vi "RTS Server Send Data.vi"(4 "Skip Data Send":bool, 6 "error in (no error)":errorcluster, 8 "error IO":errorcluster, 10 "Send Data":string[][](array[string]), 11 "TCP Network Connection in":refnum<k5>) -> (0 "error out":errorcluster, 1 "Boolean":bool, 3 "TCP Network Connection out":refnum<k5>)   [LabVIEW 2016]
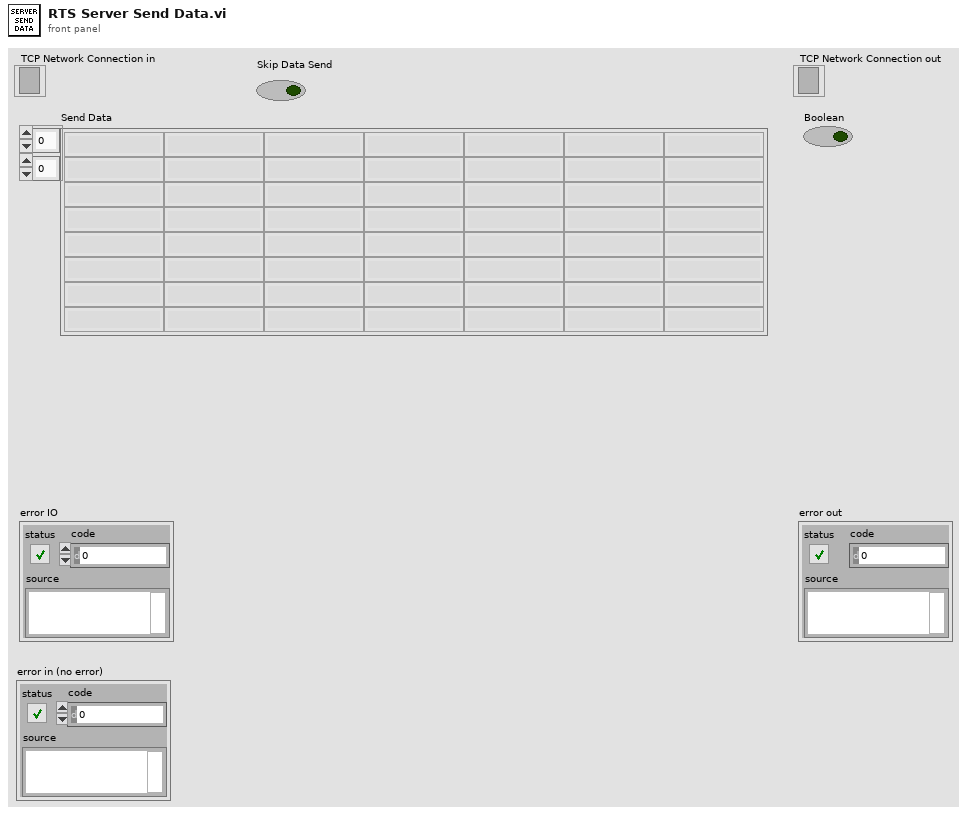
[diagram p1: front panel]
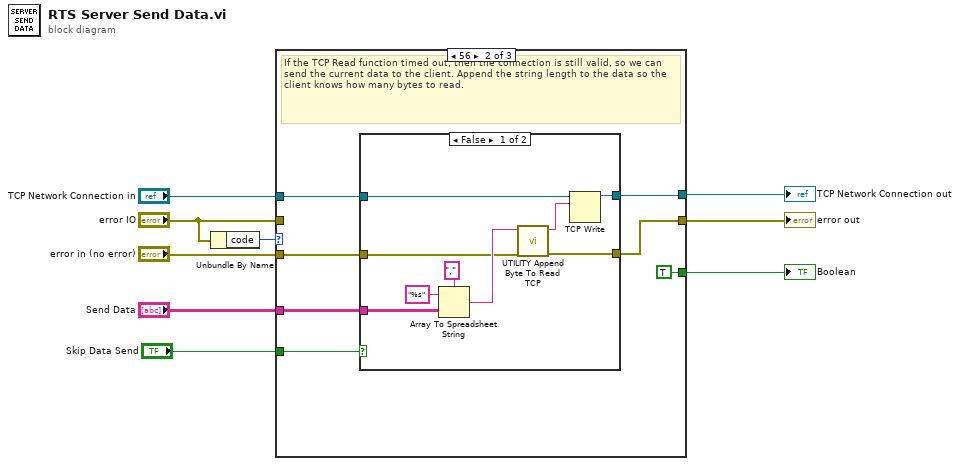
[diagram p0: block diagram]
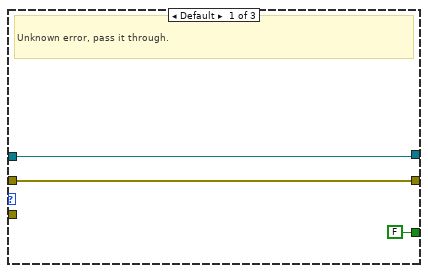
[diagram p2: hidden frame]
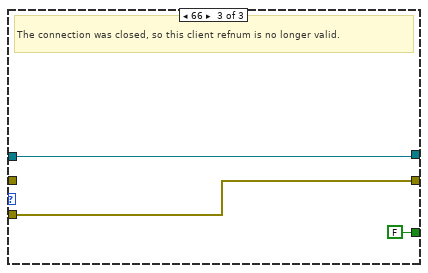
[diagram p4: hidden frame]
diagram:
  n1 = Unbundle By Name("error IO") -> ("code"=w8:i32)
  n2 = case shown="56" w8 {
    tunnel: "error IO" -> [w12 _ _]
    tunnel: [w12 w18 w33] -> w3
    tunnel: "error in (no error)" -> [_ w19 w33]
    tunnel: "TCP Network Connection in" -> [w10 w17 w31]
    tunnel: [w10 w16 w31] -> w6
    tunnel: [FALSE TRUE FALSE] -> w7
    tunnel: "Send Data" -> [_ w14 _]
    tunnel: "Skip Data Send" -> [_ w13 _]
    frame Default {
      (unwired) FALSE
      # "Unknown error, pass it through."
    }
    frame 56 {
      (unwired) TRUE
      # "If the TCP Read function timed out, then the connection is still valid, so we can send the current data to the client. Append the string length to the data so the client knows how many bytes to read."
      n3 = case shown="False" w13 {
        tunnel: w19 -> [w24 w29]
        tunnel: [w23 w29] -> w18
        tunnel: w17 -> [w22 w30]
        tunnel: [w21 w30] -> w16
        tunnel: w14 -> [w20 _]
        frame False {
          n4 = Array To Spreadsheet String(delimiter (Tab)=",", array=w20, 3:"%s" ("format string")) -> (spreadsheet string=w26:string)
          n5 = call "UTILITY Append Byte To Read TCP.vi"("Error In"=w24, "Input String"=w26) -> ("Error Out"=w23:errorcluster, "Output String"=w25:string)  [unwired: 8 in]
          n6 = TCP Write(connection ID=w22, data in=w25) -> (connection ID out=w21:refnum<k5>)  [unwired: 1 in, 3 out]
        }
        frame True {
        }
      }
    }
    frame 66 {
      (unwired) FALSE
      # "The connection was closed, so this client refnum is no longer valid."
    }
  }
  "Boolean" <- w7
  "TCP Network Connection out" <- w6
  "error out" <- w3
